vi "Form Crate Map Cluster.vi"(8 "error in":errorcluster, 11 "Display array":string[][](array[string])) -> (0 "error out":errorcluster, 2 "total channels":i32, 3 "Card Map":T1[](array[typedef]))   [LabVIEW 2018]
uses:
  card.ctl
panel:
  out "subarray":string[][](array[string])
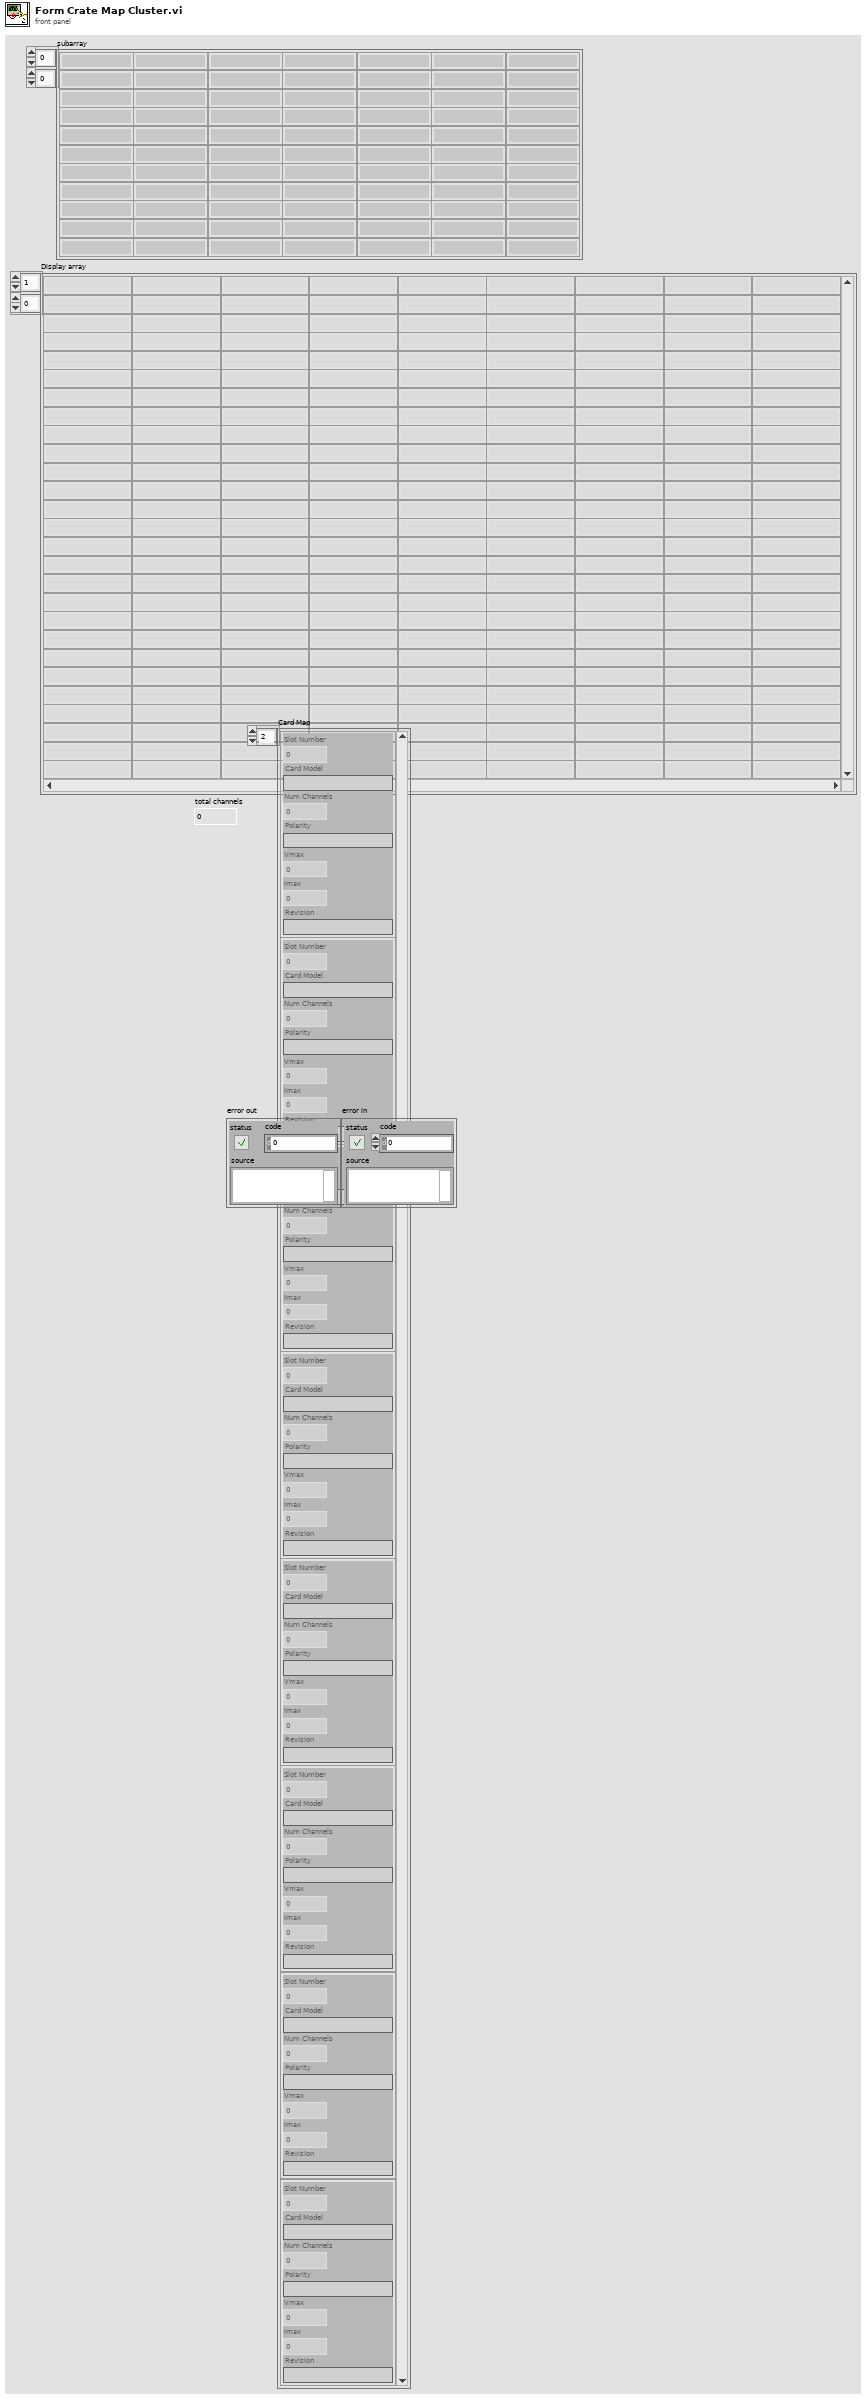
[diagram p1: front panel]
types:
  T1 = typedef "card.ctl" = cluster{"Slot Number":i32, "Card Model":string, "Num Channels":i32, "Polarity":string, "Vmax":dbl, "Imax":dbl, "Revision":string}
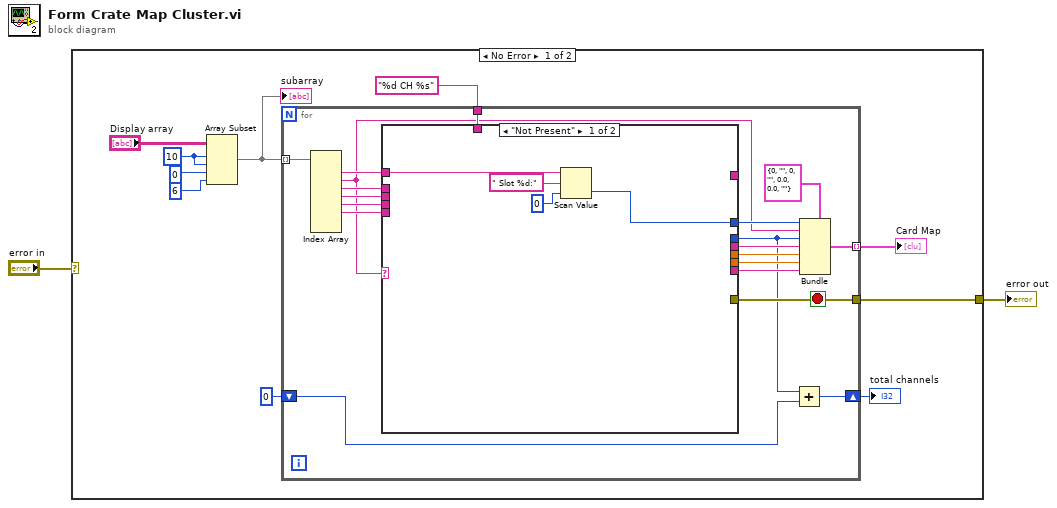
[diagram p0: block diagram]
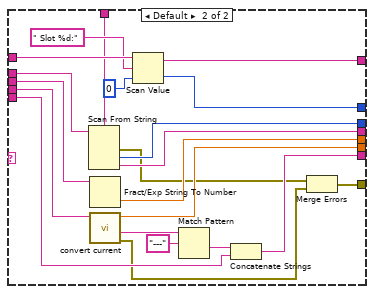
[diagram p2: hidden frame]
diagram:
  n1 = case shown="No Error" "error in" {
    selector: "error in" -> [_ w57]
    tunnel: [w6 w57] -> w2
    frame No Error {
      w12 = 10 ("index")
      n2 = Array Subset(array="Display array", index (row)=w12, length (row)=w12, index (col)=0 ("index"), length (col)=6 ("index")) -> (w8:string[][])
      "subarray" <- w8
      n3 = for {
        tunnel: w8 -> [w19] mode=indexing
        tunnel: [w21] -> w5 mode=indexing
        tunnel: "%d CH %s" ("format string") -> [w18]
        tunnel: [w16] -> w6
        shift-right: [w14] -> w3
        shift-left: 0 -> [w13]
        stop <- w16 stop-if-true
        n4 = Index Array(array=w19) -> (element #1=w31:string, element #2=w17:string, element #3=w20:string, element #4=w28:string, element #5=w26:string, element #6=w24:string)  [unwired: 8 in, 2 out]
        n5 = case shown="\"Not Present\"" w17 {
          tunnel: w31 -> [w33 w56]
          tunnel: [w32 w53] -> w30
          tunnel: [_ w52] -> w15
          tunnel: [_ w51] -> w29
          tunnel: w28 -> [_ w50]
          tunnel: [_ w49] -> w27
          tunnel: w26 -> [_ w48]
          tunnel: [_ w47] -> w25
          tunnel: w24 -> [_ w43]
          tunnel: [_ w42] -> w23
          tunnel: w20 -> [_ w41]
          tunnel: [_ w38] -> w16
          tunnel: w18 -> [_ w37]
          tunnel: [_ w36] -> _
          frame "Not Present" {
            n6 = Scan Value(string=w33, format string=" Slot %d:", default (0 dbl)=0) -> (value=w32:i32)  [unwired: 1 out]
          }
          frame Default {
            n7 = Scan From String(format string=w37, input string=w41) -> (error out=w40:errorcluster, output 1=w52:i32, output 2=w51:string)  [unwired: 4 in, 2 out]
            n8 = Fract/Exp String To Number(string=w50) -> (number=w49:dbl)  [unwired: 3 in, 1 out]
            n9 = call "convert current.vi"("input string"=w48) -> ("error IO"=w39:errorcluster, "remaining string"=w46:string, "Numeric"=w47:dbl)  [unwired: 3 in, 1 out]
            n10 = Scan Value(string=w56, format string=" Slot %d:", default (0 dbl)=0) -> (output string=w36:string, value=w53:i32)
            n11 = Match Pattern(string=w46, regular expression="---") -> (after substring=w44:string)  [unwired: 1 in, 3 out]
            n12 = Concatenate Strings(w44, w43) -> (w42:string)
            n13 = Merge Errors(w40, w39) -> (w38:errorcluster)
          }
        }
        n14 = Add(x=w15, y=w13) -> (x+y=w14:i32)
        n15 = Bundle(cluster=T1 {"Slot Number"=0, "Card Model"="", "Num Channels"=0, "Polarity"="", "Vmax"=0.0, "Imax"=0.0, "Revision"=""} ("output cluster"), "Slot Number"=w30, "Card Model"=w17, "Num Channels"=w15, "Polarity"=w29, "Vmax"=w27, "Imax"=w25, "Revision"=w23) -> (w21:T1)
      }
      "Card Map" <- w5
      "total channels" <- w3
    }
    frame Error {
    }
  }
  "error out" <- w2
